vi "FTW-Regex-Destroy.vi"(0 "Regex":refnum<data-value>, 11 "error in":errorcluster) -> (15 "error out":errorcluster)   [LabVIEW 2015]
uses:
  core/FTW-Regex-Core-Structure.ctl
panel:
  # "Inputs"
  # "Outputs"
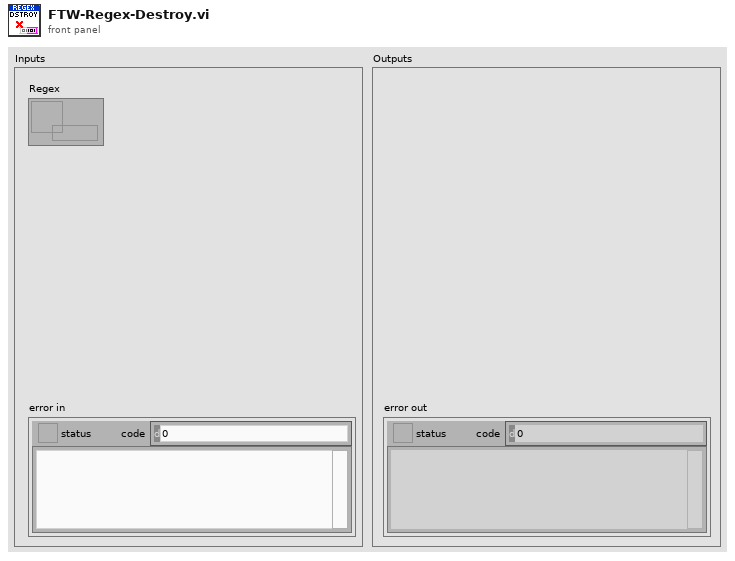
[diagram p1: front panel]
types:
  T1 = typedef "FTW-Regex-Core-Structure.ctl" = cluster{"Compiled Regex":u64}
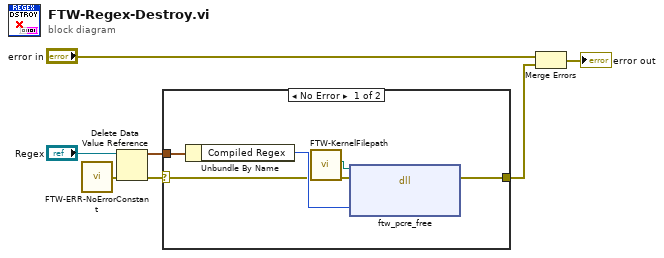
[diagram p0: block diagram]
diagram:
  n1 = call "FTW-ERR-NoErrorConstant.vi"() -> ("no error"=w3:errorcluster)
  n2 = Delete Data Value Reference(data value reference="Regex", error in=w3) -> (data value=w2:T1, error out=w1:errorcluster)
  n3 = case shown="No Error" w1 {
    selector: w1 -> [w9 _]
    tunnel: [w13 _] -> w6
    tunnel: w2 -> [w12 _]
    frame No Error {
      n4 = Unbundle By Name(w12) -> ("Compiled Regex"=w11:u64)
      n5 = call "FTW-KernelFilepath.vi"("error in"=w9) -> ("error out"=w8:errorcluster, "Library Filepath"=w10:path)  [unwired: 8 in, 1 out]
      n6 = dll-call lib="?" fn="ftw_pcre_free"(path in=w10, error in=w8, "Compiled Regex"=w11) -> (error out=w13:errorcluster)  [unwired: 3 in, 1 out]
    }
    frame Error {
    }
  }
  n7 = Merge Errors("error in", w6) -> (→"error out":errorcluster)
